vi "LabVLC - InitControl.vi"(2 "error in (no error)":errorcluster, 3 ".NET Refnum in":refnum<k24>(container), 4 "playback_video":path=path "C:/Users/admin/Desktop/BodyExplorer/VLC_LabVIEW/Ian100m10.70.mp4", 5 "vlc_dll_in":path=path "C:/Program Files (x86)/VideoLAN/VLC/libvlc.dll") -> (0 "error out":errorcluster, 1 "out":T1)   [LabVIEW 2014]
doc: "Initialize a VLC player instance. Input a video window and the path to the video. Outputs the VLC instance handle for use with the stop VI. The media pointer is passed throughout other functions. A pointer for the media player is also created but is optionally used."
uses:
  System.Windows.Forms
panel:
  out "path out":path
  out "vlc_inst_pointer":i32
  out "media_player_pointer (NC)":i32
  out "media_pointer":i32
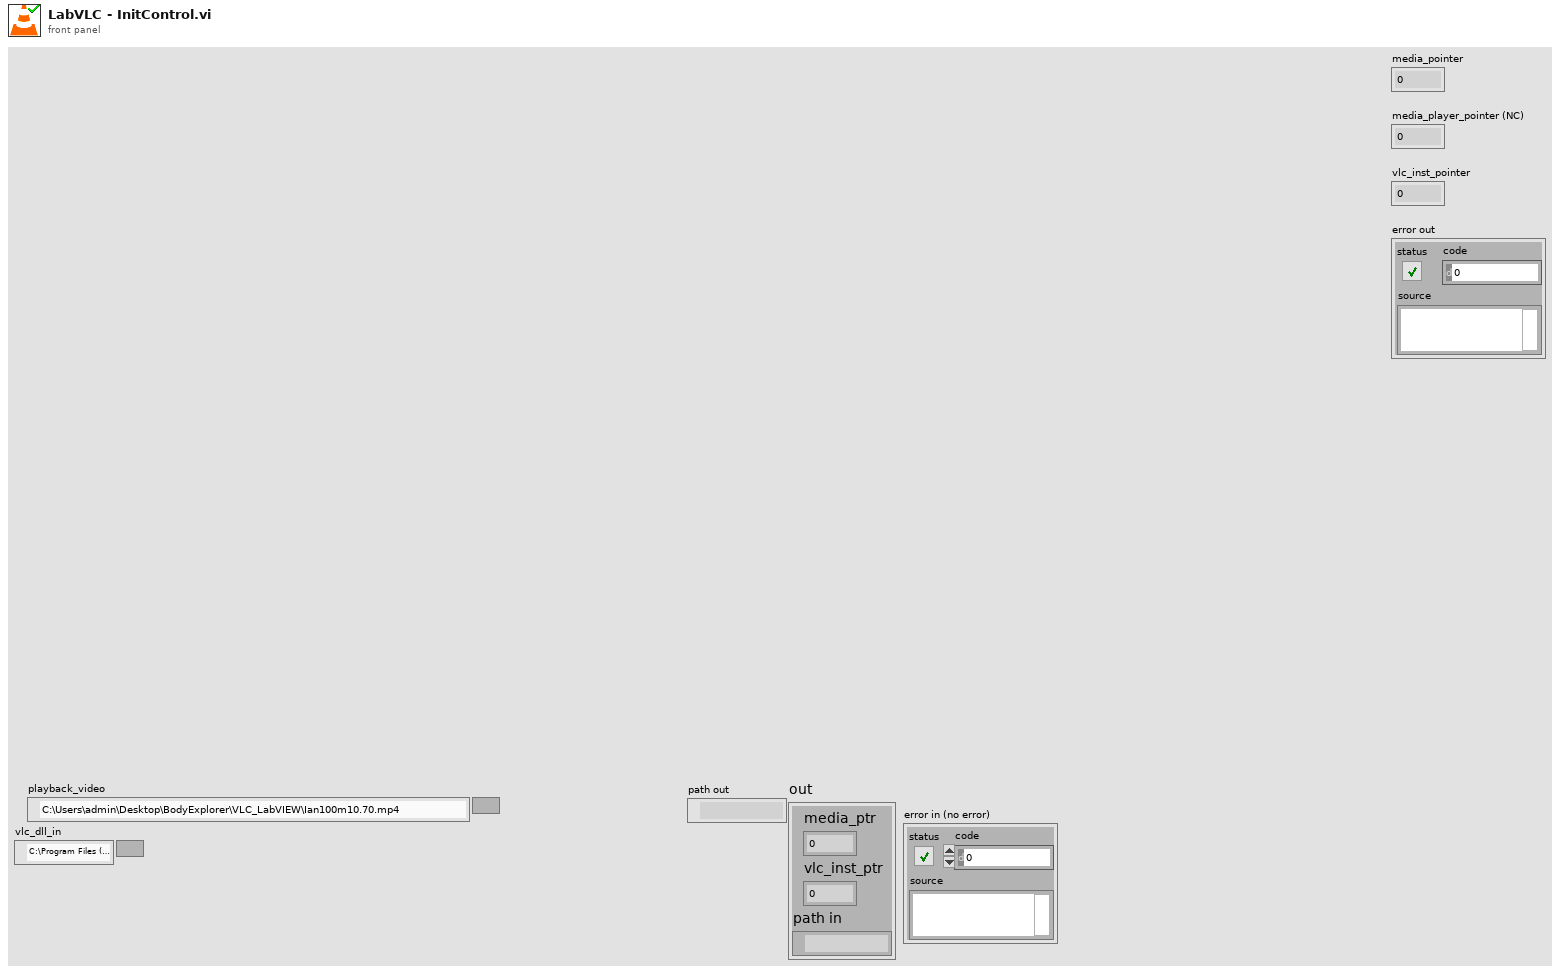
[diagram p1: front panel]
types:
  T1 = cluster{"media_ptr":i32, "vlc_inst_ptr":i32, "path in":path}
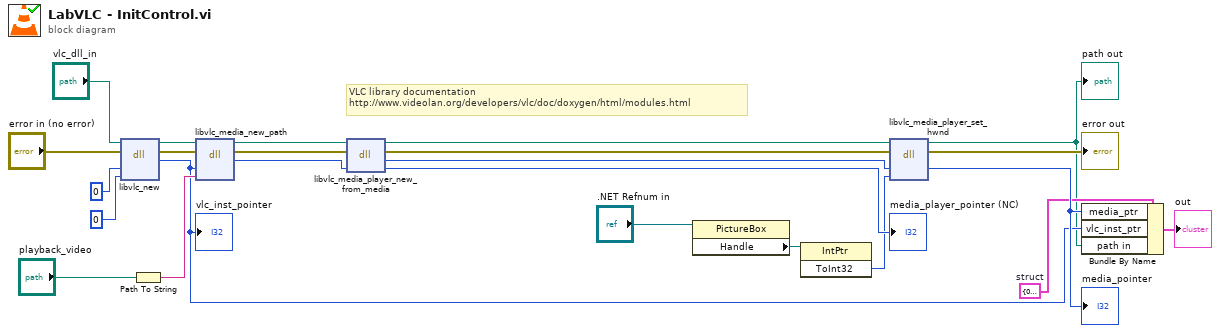
[diagram p0: block diagram]
diagram:
  w4 = T1 {"media_ptr"=0, "vlc_inst_ptr"=0, "path in"=path "C:/Program Files (x86)/VideoLAN/VLC/libvlc.dll"}  # struct
  # "VLC library documentation\nhttp://www.videolan.org/developers/vlc/doc/doxygen/html/modules.html"
  n1 = dll-call lib="C:/Program Files (x86)/VideoLAN/VLC/libvlc.dll" fn="libvlc_new"(path in="vlc_dll_in", error in="error in (no error)", "argc"=0, "argv"=u8 0) -> (path out=w9:path, error out=w11:errorcluster, "return type"=w3:i32)  [unwired: 3 in]
  "vlc_inst_pointer" <- w3
  n2 = Path To String(path="playback_video") -> (string=w19:string)
  n3 = dll-call lib="C:/Program Files (x86)/VideoLAN/VLC/libvlc.dll" fn="libvlc_media_new_path"(path in=w9, error in=w11, "p_instance"=w3, "path"=w19) -> (path out=w8:path, error out=w20:errorcluster, "return type"=w23:i32)  [unwired: 3 in]
  n4 = dll-call lib="C:/Program Files (x86)/VideoLAN/VLC/libvlc.dll" fn="libvlc_media_player_new_from_media"(path in=w8, error in=w20, "p_md"=w23) -> (path out=w7:path, error out=w12:errorcluster, "return type"=w22:i32, "p_md"=→"media_player_pointer (NC)":i32)  [unwired: 1 in]
  n5 = property class="PictureBox"(reference=".NET Refnum in") -> ("Handle"=w16:refnum<k24>)  [unwired: 1 in, 2 out]
  n6 = invoke class="IntPtr" method="ToInt32"(reference=w16) -> ("ToInt32"=w17:i32)  [unwired: 2 in, 2 out]
  n7 = dll-call lib="C:/Program Files (x86)/VideoLAN/VLC/libvlc.dll" fn="libvlc_media_player_set_hwnd"(path in=w7, error in=w12, "p_mi"=w22, "drawable"=w17) -> (path out=w2:path, error out=→"error out":errorcluster, "p_mi"=w5:i32)  [unwired: 3 in]
  "media_pointer" <- w5
  "path out" <- w2
  n8 = Bundle By Name(cluster=w4, "media_ptr"=w5, "vlc_inst_ptr"=w3, "path in"=w2) -> (→"out":T1)
